vi "Identify Oxford.vi"(8 "Error In":errorcluster, 11 "VISA resource name":refnum<visa-resource-name>) -> (0 "Error Out":errorcluster, 1 "read buffer":string, 2 "It's from Oxford!":bool, 3 "VISA resource name out":refnum<visa-resource-name>, 5 "Instrument":T1)   [LabVIEW 2019]
uses:
  Device/Device type.ctl
  Oxford crappy logic options.ctl
  GPIB/VISA  Send Receive.vi
panel:
  out "SERIAL REMAINDER":string
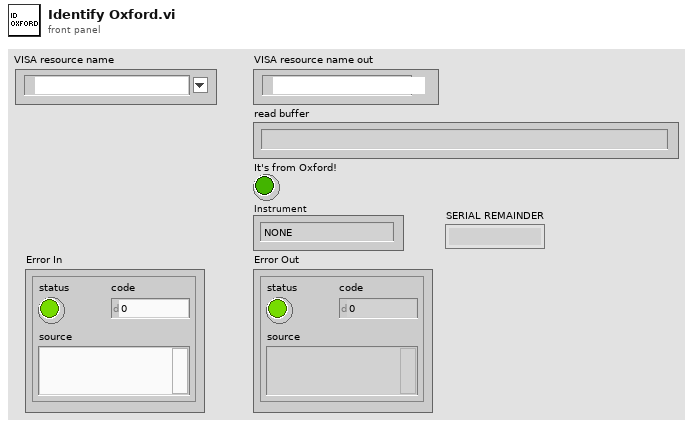
[diagram p1: front panel]
types:
  T1 = typedef "Device type.ctl" = enum16{"NONE", "Neocera 21", "LakeShore 335", "LakeShore 336", "LakeShore 340", "LkShr 340 chA&B", "LakeShore 370", "SRS 850", "SRS 830", "LR 700", "EG&G 5302", "EG&G 7260", "EG&G 7280", "AH 2500", "AH 2550", "AH 2700", "Keithley meter", "Keithley electrometer", "Keithley 182", "HP 5385", "HP 53181", "HP 53132", "ITC503", "IPS120", "Oxford Mercury IPS", "Oxford PS", "Test", "DC Facility Magnet", "Cryomagnetics PS", "Keithley 2400", "Keithley current source", "Cryo-Con 22C", "HP87NN", "HP4395A", "Agilent 34410A", "Arduino TC", "Cryo-Con 54", "Fluke 1586A"}
  T2 = typedef "Oxford crappy logic options.ctl" = enum16{"Unknown", "Serial PS", "ITC-503"}
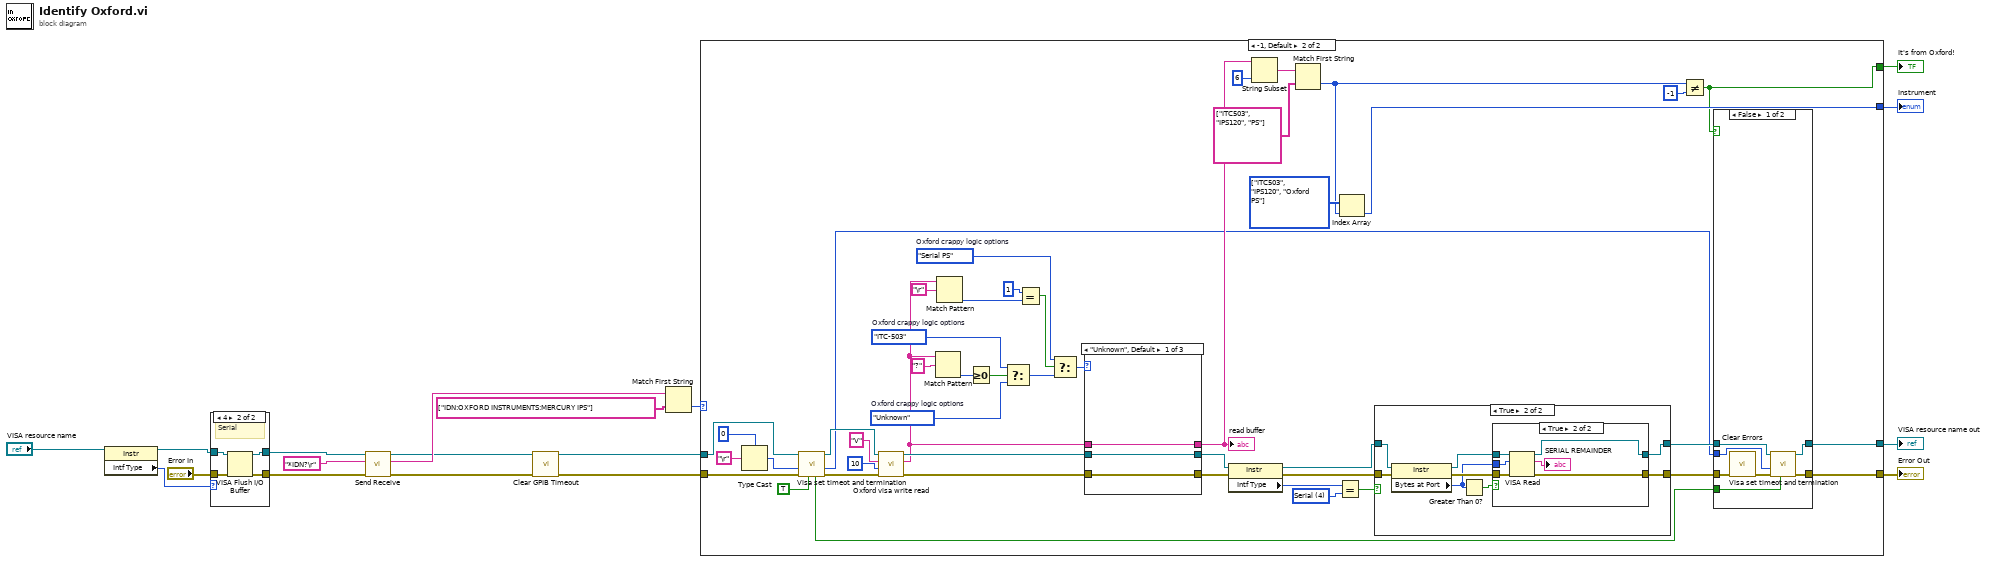
[diagram p0: block diagram]
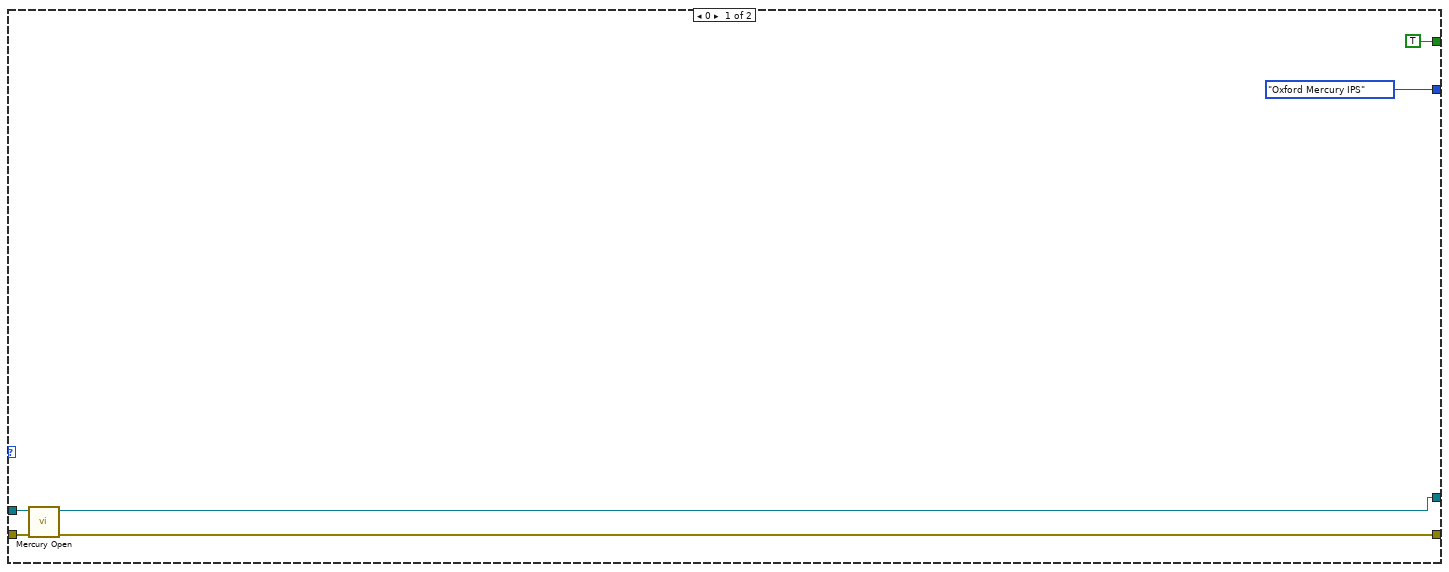
[diagram p3: hidden frame]
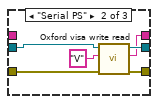
[diagram p7: hidden frame]
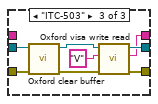
[diagram p8: hidden frame]
diagram:
  n1 = property class="Instr"(reference="VISA resource name") -> (reference out=w2:refnum<visa-resource-name>, "Intf Type"=w1:u16)  [unwired: 1 in, 1 out]
  n2 = case shown="4" w1 {
    tunnel: "Error In" -> [w18 w23]
    tunnel: [w18 w22] -> w5
    tunnel: [w19 w21] -> w4
    tunnel: w2 -> [w19 w20]
    frame 0, Default {
    }
    frame 4 {
      # "Serial"
      n3 = VISA Flush I/O Buffer(VISA resource name=w20, error in (no error)=w23) -> (VISA resource name out=w21:refnum<visa-resource-name>, error out=w22:errorcluster)  [unwired: 1 in]
    }
  }
  n4 = call-poly "Send Receive.vi"("error in (no error)"=w5, "data string in"="*IDN?\r" ("data string"), "VISA Resource Name"=w4) -> ("error out"=w13:errorcluster, "data string out"=w11:string, "VISA Resource Name Out"=w10:refnum<visa-resource-name>)  [unwired: 6 in]
  n5 = call "Clear GPIB Timeout.vi"("error in (no error)"=w13) -> ("error out"=w14:errorcluster)  [unwired: 1 in, 9 out]
  n6 = Match First String(2:string[] ["IDN:OXFORD INSTRUMENTS:MERCURY IPS"] ("string array"), 3:w11) -> (0:w8:i32)  [unwired: 1 out]
  n7 = case shown="-1, Default" w8 {
    tunnel: [w26 w33] -> w17
    tunnel: [TRUE w30] -> w16
    tunnel: [Device_type."Oxford Mercury IPS" ("Instrument") w67] -> w15
    tunnel: w14 -> [w25 w66]
    tunnel: w10 -> [w27 w65]
    tunnel: [w24 w34] -> w7
    frame 0 {
      n8 = call "Mercury Open.vi"("Error In"=w25, "VISA resource name"=w27) -> ("Error Out"=w24:errorcluster, "VISA resource name out"=w26:refnum<visa-resource-name>)  [unwired: 8 in]
    }
    frame -1, Default {
      w44 = u16 4 items=["GPIB"=1, "VXI"=2, "GPIB-VXI"=3, "Serial"=4, "PXI"=5, "TCPIP"=6, "USB"=7, "FireWire"=9] ("Interface Information:Interface Type")
      w51 = Oxford_crappy_logic_options."ITC-503"  # Oxford crappy logic options
      w53 = Oxford_crappy_logic_options."Serial PS"  # Oxford crappy logic options
      w52 = Oxford_crappy_logic_options."Unknown"  # Oxford crappy logic options
      w69 = T1[] [enum."ITC503", enum."IPS120", enum."Oxford PS"] items=["NONE", "Neocera 21", "LakeShore 335", "LakeShore 336", "LakeShore 340", "LkShr 340 chA&B", "LakeShore 370", "SRS 850", "SRS 830", "LR 700", "EG&G 5302", "EG&G 7260", "EG&G 7280", "AH 2500", "AH 2550", "AH 2700", "Keithley meter", "Keithley electrometer", "Keithley 182", "HP 5385", "HP 53181", "HP 53132", "ITC503", "IPS120", "Oxford Mercury IPS", "Oxford PS", "Test", "DC Facility Magnet", "Cryomagnetics PS", "Keithley 2400", "Keithley current source", "Cryo-Con 22C", "HP87NN", "HP4395A", "Agilent 34410A", "Arduino TC", "Cryo-Con 54", "Fluke 1586A"] ("Array")
      n9 = Type Cast(type=u8 0, x="\r") -> (*(type *) &x=w38:u8)
      n10 = call "Visa set timeot and termination.vi"("Termination Character Enable"=TRUE, "error in (no error)"=w66, "Termination Character"=w38, "VISA resource name"=w65) -> ("error out"=w74:errorcluster, "Old Termination Character"=w32:u8, "VISA resource name out"=w73:refnum<visa-resource-name>, "Old Termination Character Enable"=w31:bool)  [unwired: 3 in, 1 out]
      n11 = call "Oxford visa write read.vi"("error in (no error)"=w74, "milliseconds to wait"=u32 10, "write buffer"="V", "VISA resource name"=w73) -> ("error out"=w61:errorcluster, "read buffer"=w57:string, "VISA resource name out"=w62:refnum<visa-resource-name>)  [unwired: 5 in]
      n12 = Match Pattern(string=w57, regular expression="?") -> (offset past match=w63:i32)  [unwired: 1 in, 3 out]
      n13 = Match Pattern(string=w57, regular expression="\r") -> (offset past match=w56:i32)  [unwired: 1 in, 3 out]
      n14 = Greater Or Equal To 0?(x=w63) -> (x >= 0?=w50:bool)
      n15 = Select(t=w51, s=w50, f=w52) -> (s? t:f=w49:T2)
      n16 = Equal?(x=1, y=w56) -> (x = y?=w54:bool)
      n17 = Select(t=w53, s=w54, f=w49) -> (s? t:f=w48:T2)
      n18 = case shown="\"Unknown\", Default" w48 {
        tunnel: w62 -> [w106 w107 w120]
        tunnel: w61 -> [w105 w111 w119]
        tunnel: [w105 w110 w116] -> w60
        tunnel: [w106 w109 w114] -> w46
        tunnel: [w104 w108 w113] -> w59
        tunnel: w57 -> [w104 _ _]
        frame "Unknown", Default {
        }
        frame "Serial PS" {
          n19 = call "Oxford visa write read.vi"("error in (no error)"=w111, "write buffer"="V", "VISA resource name"=w107) -> ("error out"=w110:errorcluster, "read buffer"=w108:string, "VISA resource name out"=w109:refnum<visa-resource-name>)  [unwired: 6 in]
        }
        frame "ITC-503" {
          n20 = call "Oxford clear buffer.vi"("error in (no error)"=w119, "VISA resource name"=w120) -> ("error out"=w117:errorcluster, "VISA resource name out"=w115:refnum<visa-resource-name>)  [unwired: 6 in, 2 out]
          n21 = call "Oxford visa write read.vi"("error in (no error)"=w117, "write buffer"="V", "VISA resource name"=w115) -> ("error out"=w116:errorcluster, "read buffer"=w113:string, "VISA resource name out"=w114:refnum<visa-resource-name>)  [unwired: 6 in]
        }
      }
      "read buffer" <- w59
      n22 = property class="Instr"(reference=w46, error in=w60) -> (reference out=w42:refnum<visa-resource-name>, error out=w41:errorcluster, "Intf Type"=w45:u16)
      n23 = String Subset(string=w59, length (rest)=6 ("length (rest)")) -> (substring=w72:string)  [unwired: 1 in]
      n24 = Match First String(2:string[] ["ITC503", "IPS120", "PS"], 3:w72) -> (0:w68:i32)  [unwired: 1 out]
      n25 = Equal?(x=w45, y=w44) -> (x = y?=w43:bool)
      n26 = Index Array(array=w69, index=w68) -> (element=w67:T1)
      n27 = case shown="True" w43 {
        tunnel: w42 -> [w86 w95]
        tunnel: w41 -> [w87 w94]
        tunnel: [w86 w89] -> w36
        tunnel: [w87 w88] -> w35
        frame False {
        }
        frame True {
          n28 = property class="Instr"(reference=w95, error in=w94) -> (reference out=w93:refnum<visa-resource-name>, error out=w92:errorcluster, "Bytes at Port"=w91:u32)
          n29 = Greater Than 0?(x=w91) -> (x > 0?=w90:bool)
          n30 = case shown="True" w90 {
            tunnel: w93 -> [w96 w103]
            tunnel: w91 -> [_ w102]
            tunnel: w92 -> [w97 w101]
            tunnel: [w96 w100] -> w89
            tunnel: [w97 w99] -> w88
            frame False {
            }
            frame True {
              n31 = VISA Read(VISA resource name=w103, byte count=w102, error in (no error)=w101) -> (VISA resource name out=w100:refnum<visa-resource-name>, read buffer=→"SERIAL REMAINDER":string, error out=w99:errorcluster)  [unwired: 1 out]
            }
          }
        }
      }
      n32 = Not Equal?(x=w68, y=-1) -> (x != y?=w30:bool)
      n33 = case shown="False" w30 {
        tunnel: w35 -> [w83 w85]
        tunnel: w36 -> [w82 w84]
        tunnel: w31 -> [w80 _]
        tunnel: w32 -> [w79 _]
        tunnel: [w77 w85] -> w34
        tunnel: [w81 w84] -> w33
        frame False {
          n34 = call <vilib>:"Clear Errors.vi"("error in (no error)"=w83) -> ("error out"=w78:errorcluster)  [unwired: 5 in, 1 out]
          n35 = call "Visa set timeot and termination.vi"("Termination Character Enable"=w80, "error in (no error)"=w78, "Termination Character"=w79, "VISA resource name"=w82) -> ("error out"=w77:errorcluster, "VISA resource name out"=w81:refnum<visa-resource-name>)  [unwired: 3 in, 3 out]
        }
        frame True {
        }
      }
    }
  }
  "VISA resource name out" <- w17
  "It's from Oxford!" <- w16
  "Instrument" <- w15
  "Error Out" <- w7
